vi "20211008_01.vi"(11 "Boolean Array":bool[](array[boolean])) -> (3 "True Num.":i32)   [LabVIEW 2019]
panel:
  out ">9 Num.":i32
  in  "Numeric Array":i32[](array[numeric])
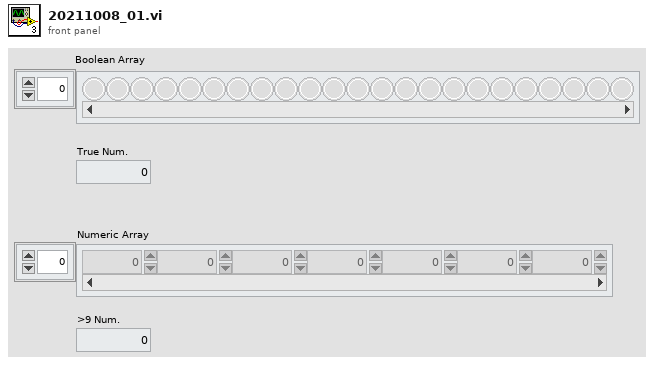
[diagram p1: front panel]
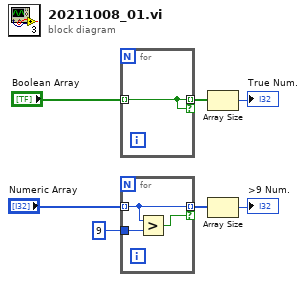
[diagram p0: block diagram]
diagram:
  n1 = for {
    tunnel: "Boolean Array" -> [w8] mode=indexing
    tunnel: [w8] -> w6 mode=indexing if=w8
  }
  n2 = for {
    tunnel: "Numeric Array" -> [w10] mode=indexing
    tunnel: [w10] -> w2 mode=indexing if=w11
    tunnel: 9 ("y") -> [w9]
    n3 = Greater?(x=w10, y=w9) -> (0:w11:bool)
  }
  n4 = Array Size(array=w6) -> (size(s)=→"True Num.":i32)
  n5 = Array Size(array=w2) -> (size(s)=→">9 Num.":i32)
